vi "Swerve Steer Cheat (SubVI).vi"(9 "Angle Error In":dbl, 11 "SteeringPower in":dbl) -> (3 "rightFrontSteeringPower out":dbl)   [LabVIEW 2020]
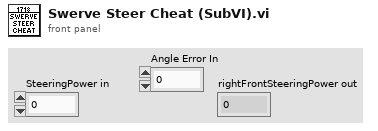
[diagram p1: front panel]
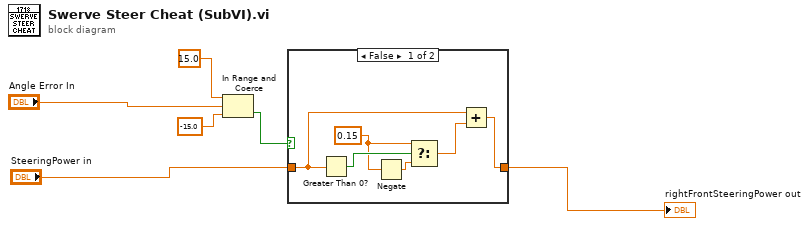
[diagram p0: block diagram]
diagram:
  n1 = In Range and Coerce(upper limit=15.0, x="Angle Error In", lower limit=-15.0) -> (In Range?=w4:bool)  [unwired: 1 out]
  n2 = case shown="False" w4 {
    tunnel: "SteeringPower in" -> [w9 w13]
    tunnel: [w7 w13] -> w6
    frame False {
      w11 = 0.15 ("t")
      n3 = Greater Than 0?(x=w9) -> (x > 0?=w12:bool)
      n4 = Negate(x=w11) -> (-x=w10:dbl)
      n5 = Select(t=w11, s=w12, f=w10) -> (s? t:f=w8:dbl)
      n6 = Add(x=w9, y=w8) -> (x+y=w7:dbl)
    }
    frame True {
    }
  }
  "rightFrontSteeringPower out" <- w6
